vi "CleanupString.vi"(1 "String":string) -> (0 "url":string)   [LabVIEW 2015]
doc: "Removes symbols from strings"
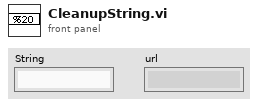
[diagram p1: front panel]
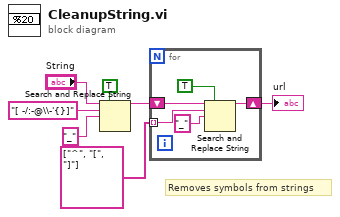
[diagram p0: block diagram]
diagram:
  # "Removes symbols from strings"
  n1 = Search and Replace String(replace all?=TRUE ("replace all? (F)"), input string="String", search string="[ -/:-@\\-'{}]", replace string="_" ("replace string (\"\")")) -> (result string=w3:string)  [unwired: 4 in, 3 out]
  n2 = for {
    tunnel: string[] ["^", "[", "]"] -> [w11] mode=indexing
    shift-right: [w9] -> w2
    shift-left: w3 -> [w10]
    n3 = Search and Replace String(replace all?=TRUE ("replace all? (F)"), input string=w10, search string=w11, replace string="_" ("replace string (\"\")")) -> (result string=w9:string)  [unwired: 4 in, 3 out]
  }
  "url" <- w2
